vi "Create (Model Files Folder).vi"(8 "error in (no error)":errorcluster, 11 "Model Files Directory":path) -> (0 "error out":errorcluster, 3 "WeChat QR Code Detector":refnum<class "WeChat QR Code Detector.lvclass">)   [LabVIEW 2020, in "feature_detection.lvlib" / "WeChat QR Code Detector.lvclass"]
doc: "Create a WeChat QR Code Detector. This uses the WeChat Object Detection and Super Resolution Neural Networks for robust QR code detection.\n\nSpecify the path of the folder which contains the detect prototxt and caffemodel as well as the sr prototxt and caffemodel files."
uses:
  WeChat QR Code Detector.lvclass
  WeChat QR Code Detector.lvclass/WeChat QR Code Detector.ctl
  Model File Paths.ctl
  a2ebe75b-f5ca-4fe5-b444-06bdc72286c0.vi
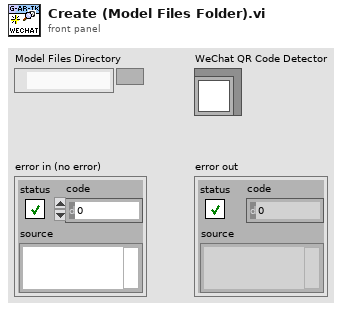
[diagram p1: front panel]
types:
  T1 = enum16{"detect.prototxt", "detect.caffemodel", "sr.prototxt", "sr.caffemodel"}
  T2 = typedef "feature_detection.lvlib/WeChat QR Code Detector.lvclass/Model File Paths.ctl" = cluster{"Detect Prototxt":path, "Detect CaffeModel":path, "SR Prototxt":path, "SR CaffeModel":path}
  T3 = enum16{"detect.prototxt", "detect.caffemodel", "sr.prototxt", "sr.caffemodel"}[]
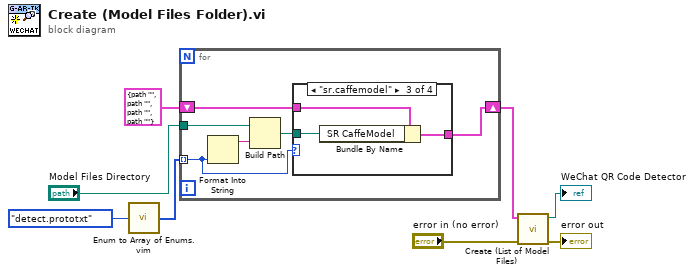
[diagram p0: block diagram]
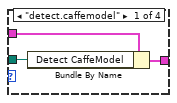
[diagram p2: hidden frame]
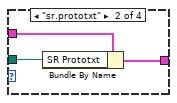
[diagram p3: hidden frame]
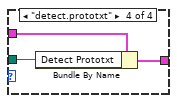
[diagram p4: hidden frame]
diagram:
  n1 = call "Enum to Array of Enums.vim"("enum"=T1."detect.prototxt") -> ("array of enums"=w3:T3)
  n2 = for {
    tunnel: w3 -> [w12] mode=indexing
    shift-right: [w10] -> w1
    shift-left: T2 {"Detect Prototxt"=path "", "Detect CaffeModel"=path "", "SR Prototxt"=path "", "SR CaffeModel"=path ""} ("Model Files") -> [w11]
    tunnel: "Model Files Directory" -> [w13]
    n3 = Format Into String(w12) -> (resulting string=w14:string)  [unwired: 3 in, 1 out]
    n4 = Build Path(base path=w13, name or relative path=w14) -> (appended path=w9:path)
    n5 = case shown="\"sr.caffemodel\"" w12 {
      tunnel: w11 -> [w16 w19 w22 w25]
      tunnel: [w17 w20 w23 w26] -> w10
      tunnel: w9 -> [w15 w18 w21 w24]
      frame "detect.caffemodel" {
        n6 = Bundle By Name(cluster=w16, "Detect CaffeModel"=w15) -> (w17:T2)
      }
      frame "sr.prototxt" {
        n7 = Bundle By Name(cluster=w19, "SR Prototxt"=w18) -> (w20:T2)
      }
      frame "sr.caffemodel" {
        n8 = Bundle By Name(cluster=w22, "SR CaffeModel"=w21) -> (w23:T2)
      }
      frame "detect.prototxt" {
        n9 = Bundle By Name(cluster=w25, "Detect Prototxt"=w24) -> (w26:T2)
      }
    }
  }
  n10 = call "Create (List of Model Files).vi"("error in (no error)"="error in (no error)", "Model Files"=w1) -> ("error out"=→"error out":errorcluster, "WeChat QR Code Detector"=→"WeChat QR Code Detector":refnum<class "WeChat QR Code Detector.lvclass">)  [unwired: 8 in]
